vi "Adjusment test - Copy_debug.vi"(2 "error in (no error)":errorcluster, 3 "Sampling rate":dbl=1000.0, 4 "Sensor":tag="SimDev1/ai0:1", 5 "VISA Refnum in":refnum<visa-resource-name>) -> (0 "error out":errorcluster, 1 "VISA Refnum out":refnum<visa-resource-name>)   [LabVIEW 2020]
uses:
  <vilib>/DAQmx/read.llb/DAQmx Read (Analog 1D DBL NChan 1Samp).vi
  <vilib>/DAQmx/create/channels.llb/DAQmx Create Channel (AI-Voltage-Basic).vi
  <vilib>/DAQmx/configure/timing.llb/DAQmx Timing (Sample Clock).vi
  <vilib>/DAQmx/miscellaneous.llb/DAQmx Fill In Error Info.vi
panel:
  out "Force Sensor":dbl
  out "Precise Sensor":dbl
  out "Changing Weg":dbl
  in  "Lower limit for position":dbl
  in  "Upper limit for position":dbl
  in  "Up":bool
  out "State":u32
  in  "Stop":bool
  in  "Down":bool
  in  "Speed":bool
  in  "maschine Version":bool
  in  "Speed Write in micrometer/sec":string
  out "Standard output":string
  out "Numeric 3":i32
  in  "Exit Program":bool
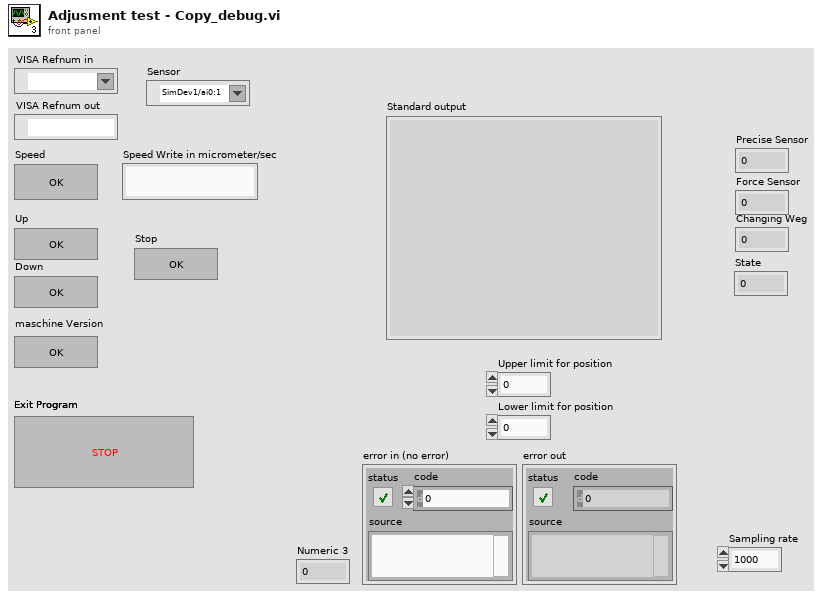
[diagram p1: front panel]
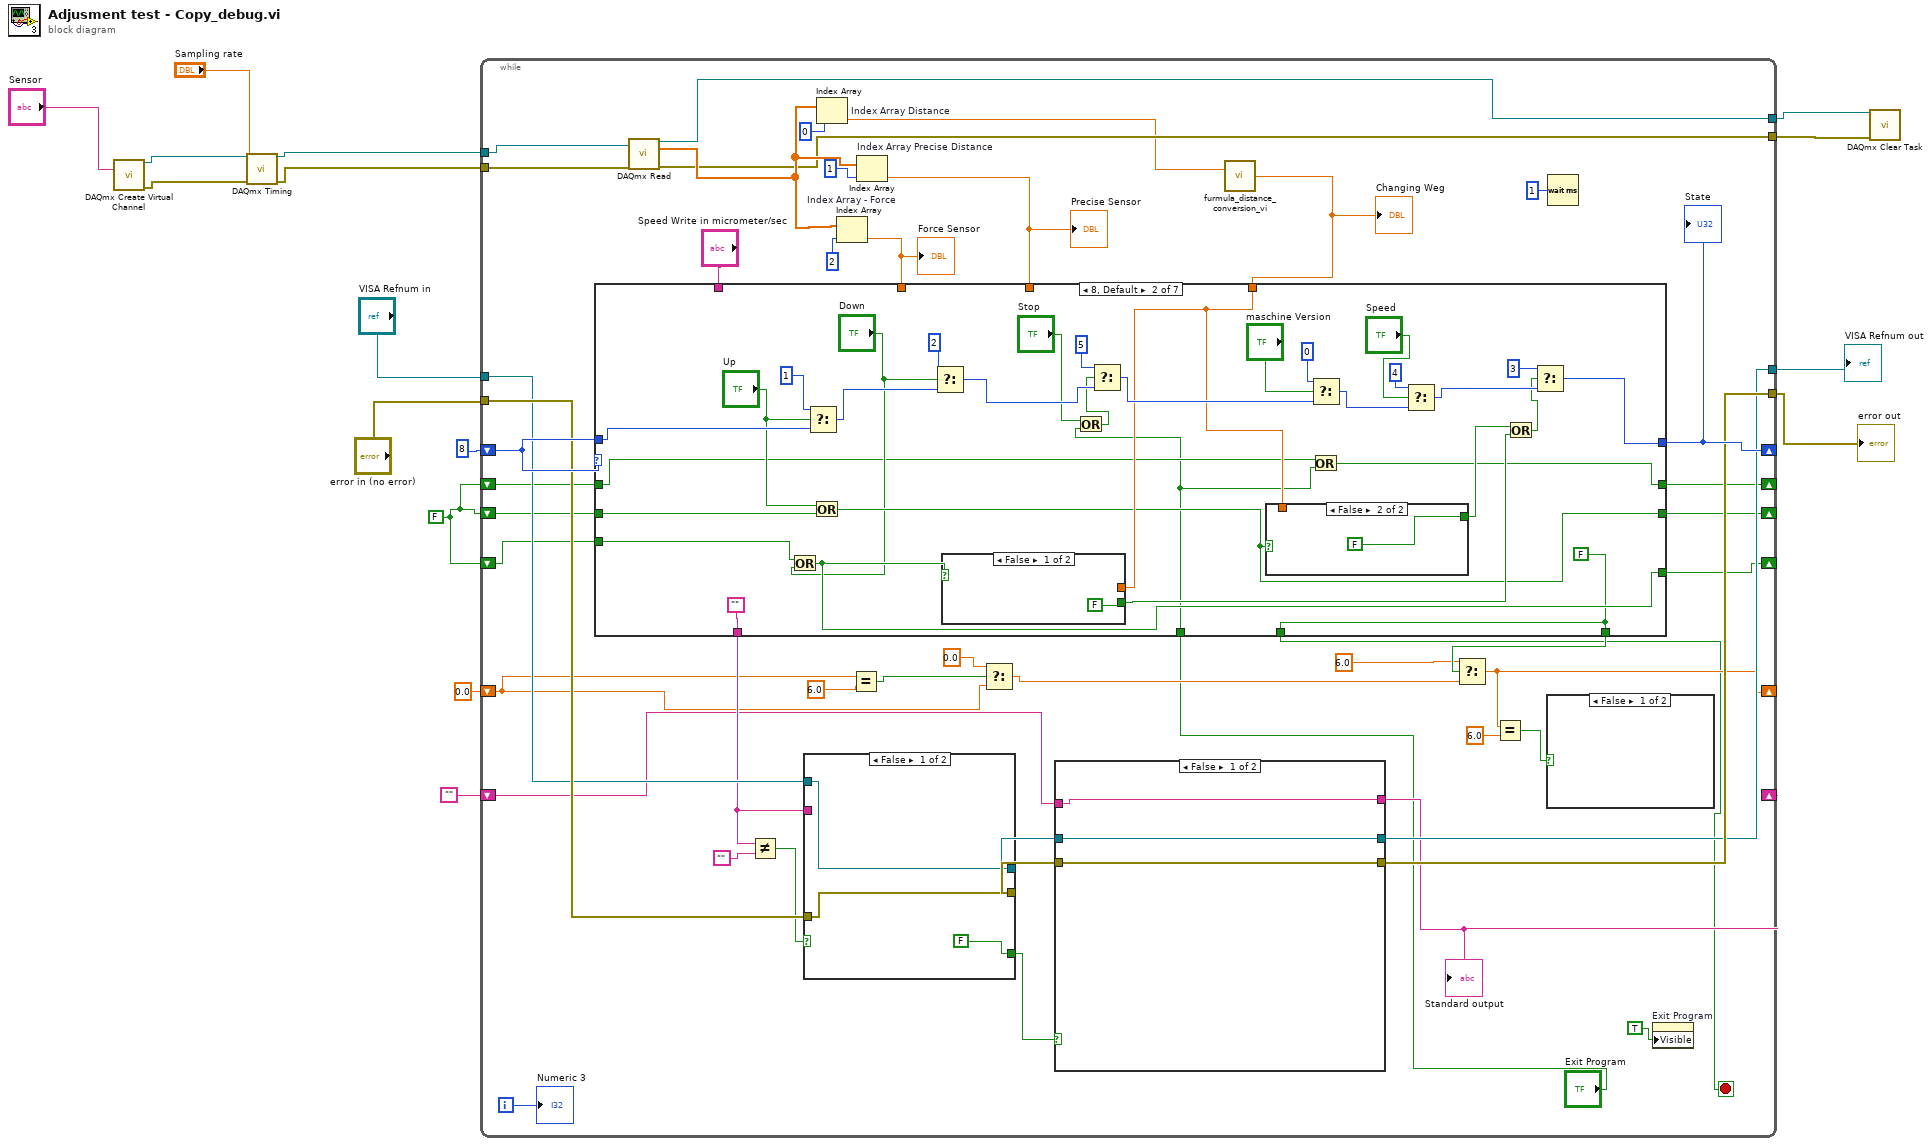
[diagram p0: block diagram]
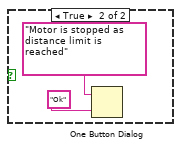
[diagram p2: hidden frame]
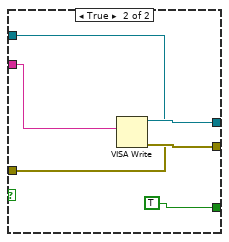
[diagram p3: hidden frame]
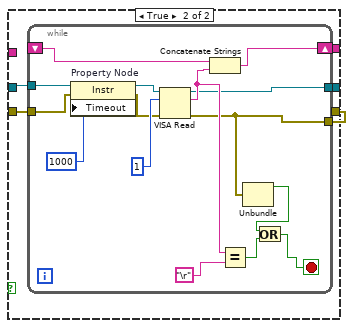
[diagram p4: hidden frame]
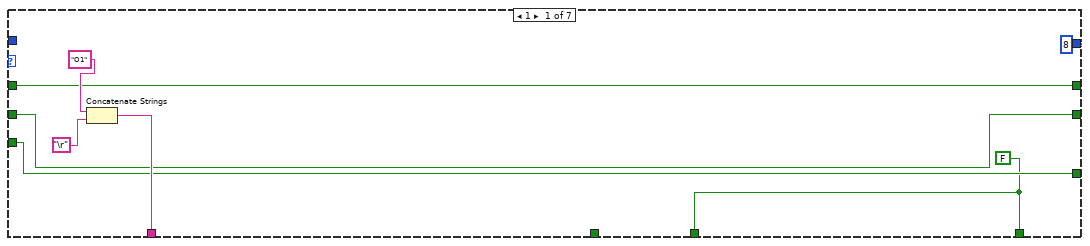
[diagram p5: hidden frame]
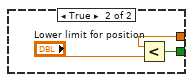
[diagram p6: hidden frame]
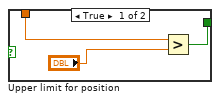
[diagram p7: hidden frame]
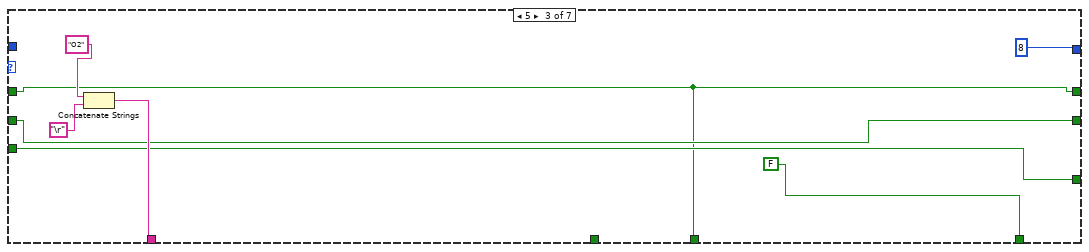
[diagram p8: hidden frame]
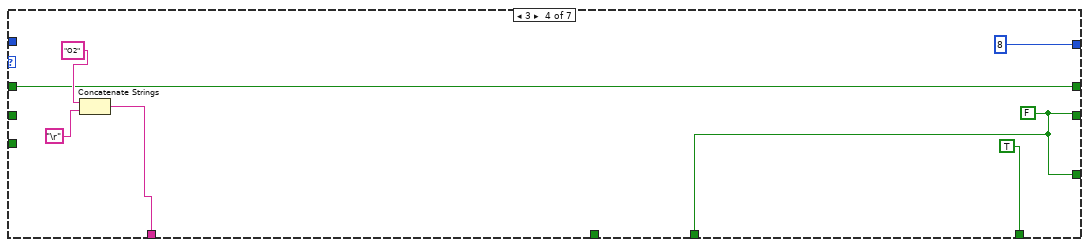
[diagram p9: hidden frame]
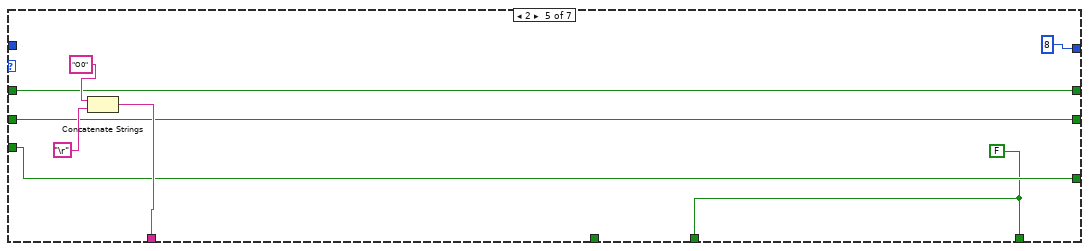
[diagram p10: hidden frame]
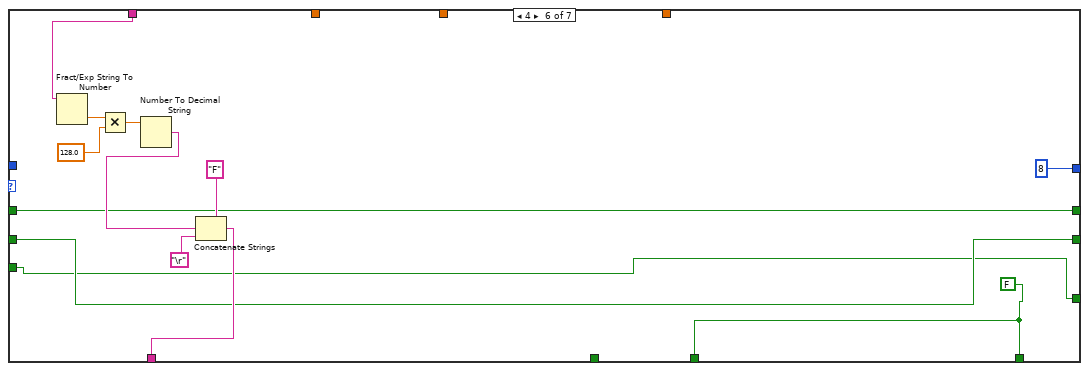
[diagram p11: hidden frame]
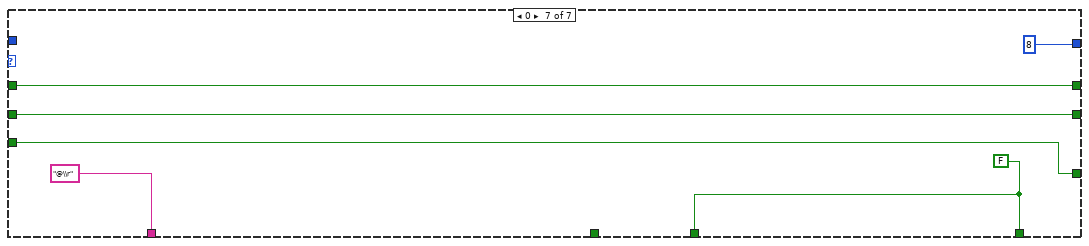
[diagram p12: hidden frame]
diagram:
  w1 = FALSE
  n1 = call-poly <vilib>:"DAQmx Create Virtual Channel.vi"("physical channels"="Sensor") -> ("task out"=w10:refnum<k21>, "error out"=w9:errorcluster)  [unwired: 13 in]
  n2 = call-poly <vilib>:"DAQmx Timing.vi"("task/channels in"=w10, "rate"="Sampling rate", "error in"=w9) -> ("task out"=w6:refnum<k21>, "error out"=w5:errorcluster)  [unwired: 11 in]
  n3 = while {
    tunnel: "VISA Refnum in" -> [w55]
    tunnel: "error in (no error)" -> [w56]
    tunnel: [w59] -> w14
    tunnel: [w58] -> w15
    shift-right: [w63] -> _
    shift-left: 8 -> [w57]
    shift-right: [w50] -> _
    shift-left: "" -> [w49]
    tunnel: w6 -> [w48]
    tunnel: w5 -> [w47]
    tunnel: [w40] -> w4
    tunnel: [w39] -> w3
    shift-right: [w36] -> _
    shift-left: 0.0 ("t") -> [w30]
    shift-right: [w27] -> _
    shift-left: w1 -> [w26]
    shift-right: [w24] -> _
    shift-left: w1 -> [w25]
    shift-right: [w19] -> _
    shift-left: w1 -> [w18]
    i -> [w64]
    stop <- w17 stop-if-true
    n4 = call-poly <vilib>:"DAQmx Read.vi"("task/channels in"=w48, "error in"=w47) -> ("task out"=w40:refnum<k21>, "data"=w43:dbl[], "error out"=w39:errorcluster)  [unwired: 11 in]
    n5 = Index Array "Index Array Distance"(array=w43, index=0) -> (element=w22:dbl)
    n6 = Index Array "Index Array - Force"(array=w43, index=2) -> (element=w42:dbl)
    "Force Sensor" <- w42
    n7 = Equal?(x=w30, y=6.0) -> (x = y?=w32:bool)
    n8 = Index Array "Index Array Precise Distance"(array=w43, index=1) -> (element=w41:dbl)
    "Precise Sensor" <- w41
    n9 = Select(t=0.0, s=w32, f=w30) -> (s? t:f=w29:dbl)
    n10 = call "furmula_distance_conversion_vi.vi"("Schieberegler"=w22) -> ("Numeric"=w23:dbl)
    "Changing Weg" <- w23
    n11 = case shown="8, Default" w57 {
      tunnel: [8 w124 8 8 8 u32 8 ("byte count") 8] -> w63
      tunnel: [w104 "" w152 w159 w167 w175 "@\\r" ("write buffer")] -> w53
      tunnel: w57 -> [_ w138 _ _ _ _ _]
      tunnel: "Speed Write in micrometer/sec" -> [_ _ _ _ _ w177 _]
      tunnel: w23 -> [_ w127 _ _ _ _ _]
      tunnel: w42 -> [_ _ _ _ _ _ _]
      tunnel: w41 -> [_ _ _ _ _ _ _]
      tunnel: [w99 w107 FALSE TRUE w163 w171 w184] -> w38
      tunnel: [w102 w117 w150 w156 w165 w173 w186] -> w27
      tunnel: w26 -> [w102 w118 w150 _ w165 w173 w186]
      tunnel: w25 -> [w101 w116 w149 _ w164 w172 w185]
      tunnel: [w101 w115 w149 w156 w164 w172 w185] -> w24
      tunnel: "Exit Program" -> [_ w109 _ _ _ _ _]
      tunnel: [w100 w108 w147 w155 w162 w170 w183] -> w19
      tunnel: w18 -> [w100 w110 w147 w155 w162 w170 w183]
      tunnel: [w99 w107 w147 w156 w163 w171 w184] -> w17
      frame 1 {
        w99 = FALSE
        n12 = Concatenate Strings("O1", "\r") -> (w104:string)
      }
      frame 8, Default {
        w107 = FALSE
        n13 = Or(x=w116, y="Down") -> (x .or. y?=w115:bool)
        n14 = Select(t=u32 1, s="Up", f=w138) -> (s? t:f=w120:u32)
        n15 = Or(x="Up", y=w118) -> (x .or. y?=w117:bool)
        n16 = Select(t=u32 2, s="Down", f=w120) -> (s? t:f=w130:u32)
        n17 = case shown="False" w115 {
          tunnel: w127 -> [_ w142]
          tunnel: [FALSE w141] -> w119
          frame False {
          }
          frame True {
            n18 = Less?(x=w142, y="Lower limit for position") -> (x < y?=w141:bool)
          }
        }
        n19 = Or(x="Stop", y=w109) -> (x .or. y?=w111:bool)
        n20 = Select(t=u32 5, s=w111, f=w130) -> (s? t:f=w129:u32)
        n21 = case shown="False" w117 {
          tunnel: w127 -> [w144 _]
          tunnel: [w143 FALSE] -> w126
          frame True {
            n22 = Greater?(x=w144, y="Upper limit for position") -> (0:w143:bool)
          }
          frame False {
          }
        }
        n23 = Select(t=0, s="maschine Version", f=w129) -> (s? t:f=w132:u32)
        n24 = Or(x=w110, y=w109) -> (x .or. y?=w108:bool)
        n25 = Select(t=4, s="Speed", f=w132) -> (s? t:f=w125:u32)
        n26 = Or(x=w126, y=w119) -> (x .or. y?=w122:bool)
        n27 = Select(t=u32 3, s=w122, f=w125) -> (s? t:f=w124:u32)
      }
      frame 5 {
        n28 = Concatenate Strings("O2", "\r") -> (w152:string)
      }
      frame 3 {
        w156 = FALSE
        n29 = Concatenate Strings("O2", "\r") -> (w159:string)
      }
      frame 2 {
        w163 = FALSE
        n30 = Concatenate Strings("O0", "\r") -> (w167:string)
      }
      frame 4 {
        w171 = FALSE
        n31 = Fract/Exp String To Number(string=w177) -> (number=w180:dbl)  [unwired: 3 in, 1 out]
        n32 = Multiply(x=w180, y=128.0) -> (x*y=w181:dbl)
        n33 = Number To Decimal String(number=w181) -> (decimal integer string=w176:string)  [unwired: 1 in]
        n34 = Concatenate Strings("F", w176, "\r") -> (w175:string)
      }
      frame 0 {
        w184 = FALSE
      }
    }
    "State" <- w63
    n35 = Not Equal?(x=w53, y="") -> (x != y?=w52:bool)
    n36 = case shown="False" w52 {
      tunnel: [FALSE TRUE] -> w60
      tunnel: [w68 w73] -> w61
      tunnel: [w67 w74] -> w62
      tunnel: w53 -> [_ w70]
      tunnel: w56 -> [w67 w72]
      tunnel: w55 -> [w68 w71]
      frame False {
      }
      frame True {
        n37 = VISA Write(VISA resource name=w71, write buffer=w70, error in (no error)=w72) -> (VISA resource name out=w73:refnum<visa-resource-name>, error out=w74:errorcluster)  [unwired: 1 out]
      }
    }
    n38 = case shown="False" w60 {
      tunnel: [w77 w79] -> w59
      tunnel: [w78 w80] -> w58
      tunnel: [w76 w83] -> w50
      tunnel: w61 -> [w78 w81]
      tunnel: w62 -> [w77 w82]
      tunnel: w49 -> [w76 _]
      frame False {
      }
      frame True {
        n39 = while {
          shift-right: [w96] -> w83
          shift-left: _ -> [w97]
          tunnel: w82 -> [w87]
          tunnel: w81 -> [w86]
          tunnel: [w85] -> w80
          tunnel: [w84] -> w79
          stop <- w92 stop-if-true
          n40 = property on="Property Node" class="Instr"(reference=w86, error in=w87, "Timeout"=u32 1000 ("General Settings:Timeout Value")) -> (reference out=w91:refnum<visa-resource-name>, error out=w90:errorcluster)
          n41 = VISA Read(VISA resource name=w91, byte count=u32 1, error in (no error)=w90) -> (VISA resource name out=w85:refnum<visa-resource-name>, read buffer=w95:string, error out=w84:errorcluster)  [unwired: 1 out]
          n42 = Concatenate Strings(w97, w95) -> (w96:string)
          n43 = Equal?(x=w95, y="\r") -> (x = y?=w93:bool)
          n44 = Unbundle(w84) -> ("status"=w88:bool)  [unwired: 2 out]
          n45 = Or(x=w88, y=w93) -> (x .or. y?=w92:bool)
        }
      }
    }
    "Standard output" <- w50
    n46 = Select(t=6.0, s=w38, f=w29) -> (s? t:f=w36:dbl)
    n47 = Equal?(x=w36, y=6.0) -> (x = y?=w34:bool)
    n48 = case shown="False" w34 {
      frame False {
      }
      frame True {
        n49 = One Button Dialog(message="Motor is stopped as  distance limit is reached", button name ("OK")="Ok") -> ()  [unwired: 1 out]
      }
    }
    n50 = Wait (ms)(milliseconds to wait=u32 1) -> ()  [unwired: 1 out]
    n51 = property on="Exit Program" class="Bool"("Visible"=TRUE) -> ()  [unwired: 2 in, 2 out]
    "Numeric 3" <- w64
  }
  "VISA Refnum out" <- w15
  "error out" <- w14
  n52 = call <vilib>:"DAQmx Clear Task.vi"("task in"=w4, "error in"=w3) -> ()  [unwired: 13 in, 1 out]
